vi "ClustersToIni.vi"(8 "ErrorArray in":errorcluster[](array[cluster]), 10 "ClusterRefArray":refnum<vi>[](array[refnum]), 11 "IniFileRef in":T1) -> (0 "ErrorArray out":errorcluster[](array[cluster]), 3 "IniFileRef out":T1)   [LabVIEW 2014, in "Ini_lib.lvlib"]
uses:
  Ini_lib.lvlib
  <vilib>/Utility/config.llb/Config Data RefNum.ctl
  <userlib>/NIST/NISTErrorLib/NISTErrorLib.lvlib
  <vilib>/Utility/config.llb/NI_LVConfig.lvlib
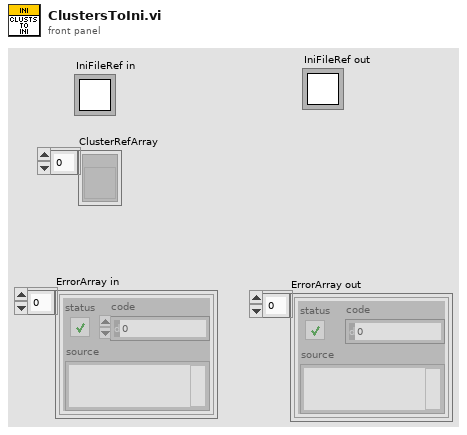
[diagram p1: front panel]
types:
  T1 = typedef "NI_LVConfig.lvlib/Config Data RefNum.ctl" = refnum<k1>
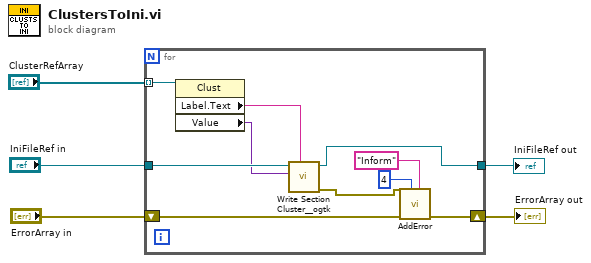
[diagram p0: block diagram]
diagram:
  n1 = for {
    tunnel: "ClusterRefArray" -> [w15] mode=indexing
    tunnel: "IniFileRef in" -> [w14]
    shift-right: [w11] -> w1
    shift-left: "ErrorArray in" -> [w7]
    tunnel: [w6] -> w2
    n2 = property class="Clust"(reference=w15) -> ("Label.Text"=w13:string, "Value"=w12:variant)  [unwired: 1 in, 2 out]
    n3 = call <userlib>:"Write Section Cluster__ogtk.vi"("section (optional)"=w13, "Section Formatted Cluster"=w12, "refnum"=w14) -> ("error out"=w8:errorcluster, "dup refnum"=w6:T1)  [unwired: 7 in]
    n4 = call <userlib>:"AddError.vi"("Severity"="Inform", "Priority"=u8 4, "ErrorArray"=w7, "error in (no error)"=w8) -> ("ErrorArray"=w11:errorcluster[])  [unwired: 6 in, 1 out]
  }
  "ErrorArray out" <- w1
  "IniFileRef out" <- w2
